vi "GT_EncSns.vi"(2 "Sense":u16, 3 "rtn_In":cluster{"rtn":i16, "Func":string}) -> (1 "rtn_Out":cluster{"rtn":i16, "Func":string})   [LabVIEW 2014]
uses:
  VC6/gts.dll
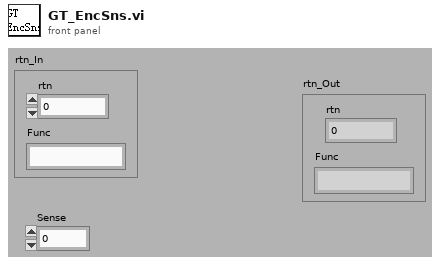
[diagram p1: front panel]
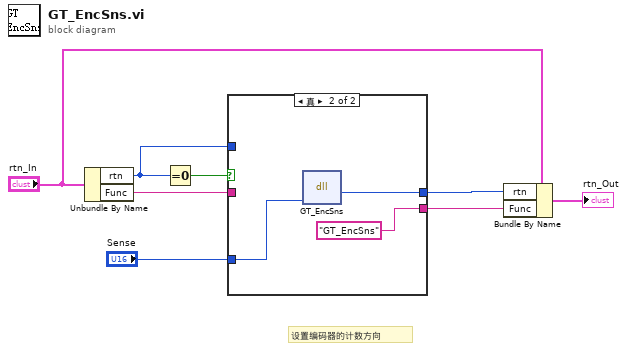
[diagram p0: block diagram]
diagram:
  # "设置编码器的计数方向"
  n1 = Unbundle By Name("rtn_In") -> ("rtn"=w1:i16, "Func"=w7:string)
  n2 = Equal To 0?(x=w1) -> (x = 0?=w8:bool)
  n3 = case shown="真" w8 {
    tunnel: w7 -> [w9 _]
    tunnel: "Sense" -> [_ w13]
    tunnel: [w10 w12] -> w4
    tunnel: [w9 "GT_EncSns" ("Func")] -> w3
    tunnel: w1 -> [w10 _]
    frame False {
    }
    frame True {
      n4 = dll-call lib="PTH2Fabs DNewGTS AC-800LWin7版源程序-20170926gts85VC6gts.dll" fn="GT_EncSns"("Sense"=w13) -> ("rtn"=w12:i16)  [unwired: 4 in, 2 out]
    }
  }
  n5 = Bundle By Name(cluster="rtn_In", "rtn"=w4, "Func"=w3) -> (→"rtn_Out":cluster{"rtn":i16, "Func":string})
